vi "poumianS.vi"(0 "object in":refnum<class "212format_work.lvclass">, 1 "in":T2, 5 "error in (no error)":errorcluster) -> (14 "object out":refnum<class "212format_work.lvclass">, 15 "out":T1, 19 "error out":errorcluster)   [LabVIEW 2016, in "212format_work.lvclass"]
uses:
  212format_work.lvclass
  212format_work.lvclass/212format_work.ctl
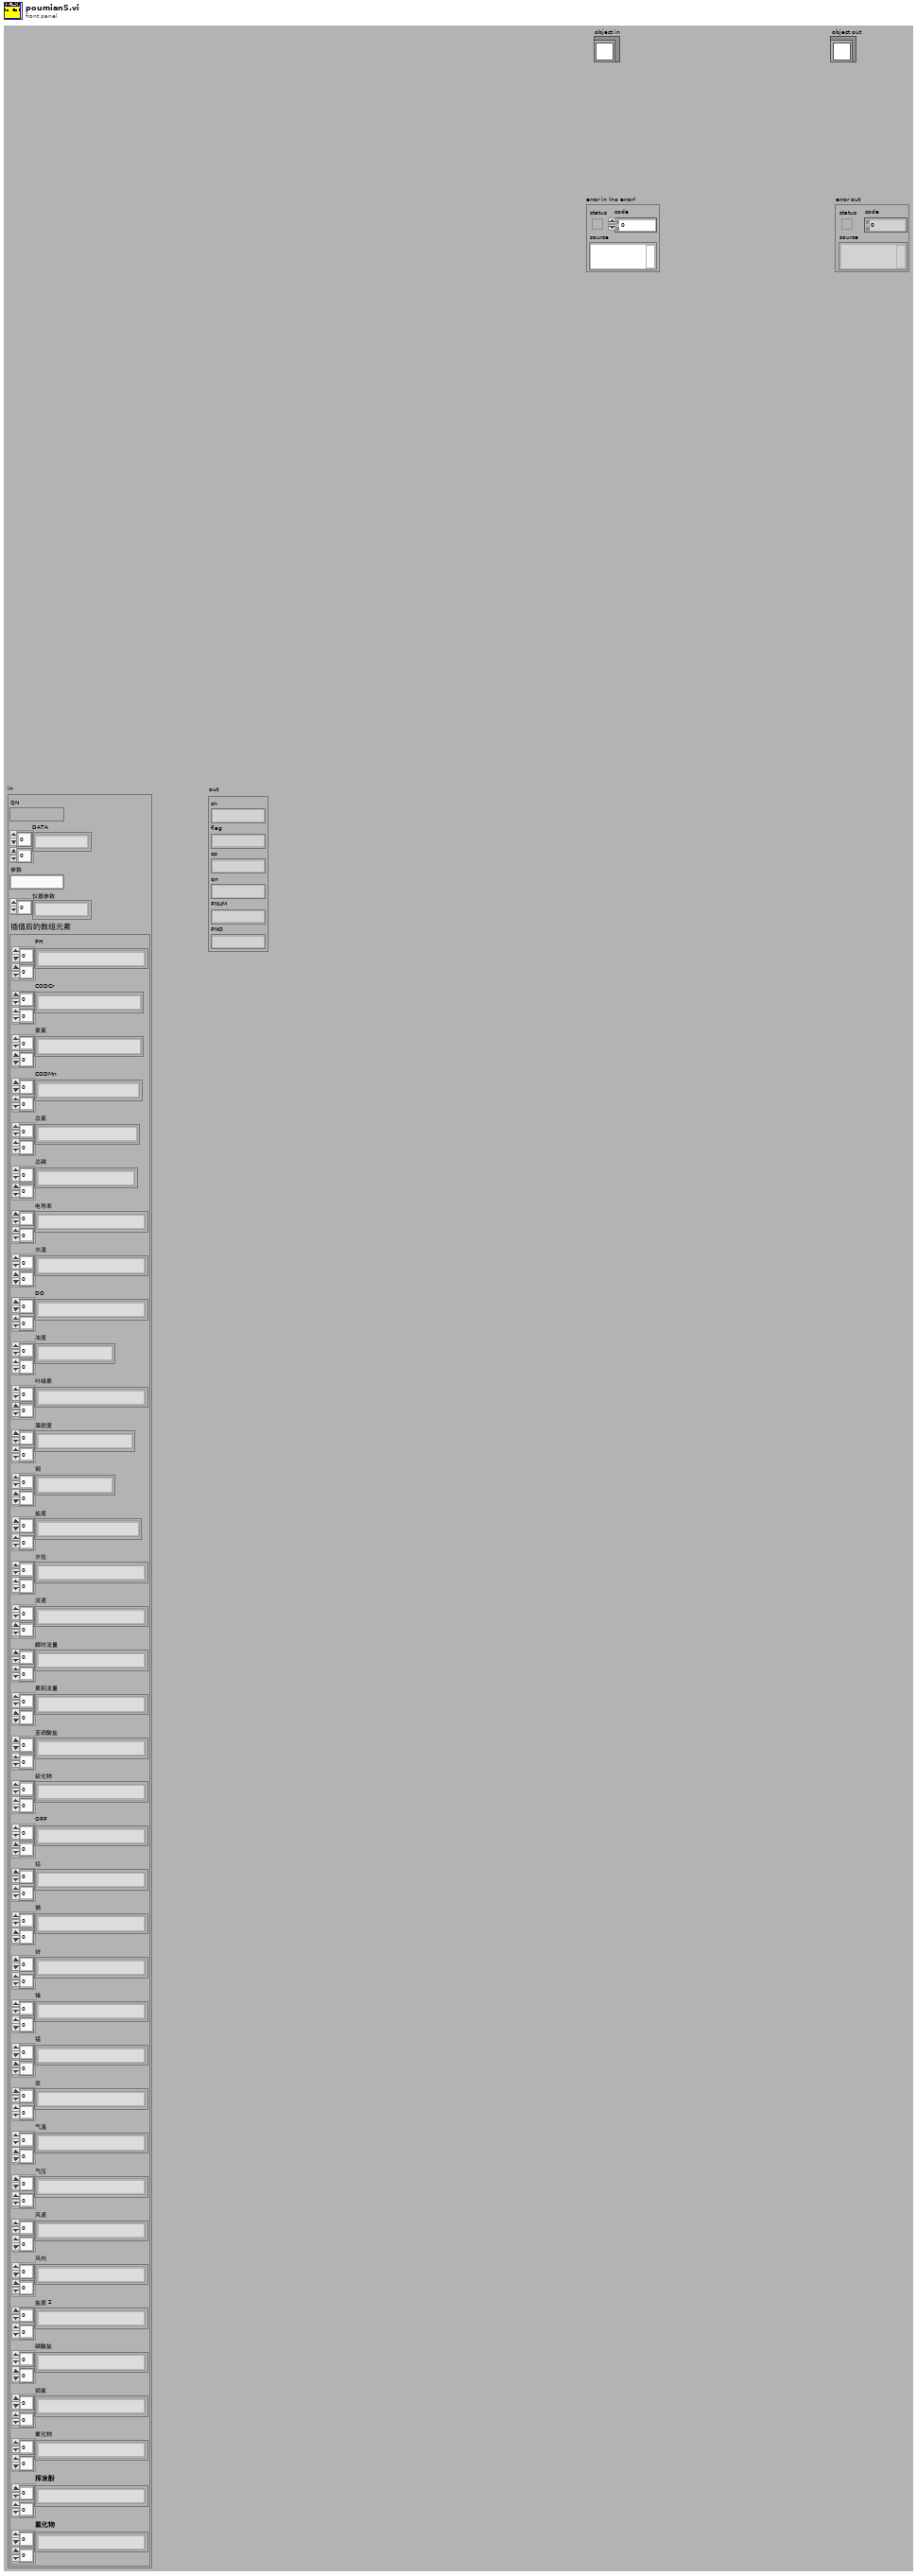
[diagram p1: front panel]
types:
  T1 = cluster{"cn":string, "flag":string, "cp":string, "qn":string, "PNUM":string, "PNO":string}
  T2 = cluster{"QN":string, "DATA":string[][], "参数":string, "仪器参数":string[], "插值后的数组元素":cluster{"PH":string[][], "CODCr":string[][], "氨氮":string[][], "CODMn":string[][], "总氮":string[][], "总磷":string[][], "电导率":string[][], "水温":string[][], "DO":string[][], "浊度":string[][], "叶绿素":string[][], "藻密度":string[][], "铜":string[][], "盐度":string[][], "水位":string[][], "流速":string[][], "瞬时流量":string[][], "累积流量":string[][], "亚硝酸盐":string[][], "硫化物":string[][], "ORP":string[][], "铅":string[][], "镉":string[][], "锌":string[][], "镍":string[][], "锰":string[][], "汞":string[][], "气温":string[][], "气压":string[][], "风速":string[][], "风向":string[][], "盐度 2":string[][], "磷酸盐":string[][], "硝氮":string[][], "氟化物":string[][], "挥发酚":string[][], "氯化物":string[][]}}
  T3 = enum16{"formattime", "formatminute", "formathour"}
  T4 = typedef "212format_work.lvclass/interdata控件.ctl" = cluster{"数据发送协议":enum16{"2005-212协议", "2017-212协议"}, "枚举":enum16{"返回请求应答", "上传数据", "返回执行结果"}, "系统编码ST":string, "主动上报数据中":bool, "数据组合发送":bool, "地表水/污染源":bool, "应用环境":enum16{"STD", "GB212"}}
  T5 = typedef "212format_work.lvclass/data控件.ctl" = cluster{"选择发送的参数":string, "插值后的数组元素":cluster{"PH":string[][], "CODCr":string[][], "氨氮":string[][], "CODMn":string[][], "总氮":string[][], "总磷":string[][], "电导率":string[][], "水温":string[][], "DO":string[][], "浊度":string[][], "叶绿素":string[][], "藻密度":string[][], "铜":string[][], "盐度":string[][], "水位":string[][], "流速":string[][], "瞬时流量":string[][], "累积流量":string[][], "亚硝酸盐":string[][], "硫化物":string[][], "ORP":string[][], "铅":string[][], "镉":string[][], "锌":string[][], "镍":string[][], "锰":string[][], "汞":string[][], "气温":string[][], "气压":string[][], "风速":string[][], "风向":string[][], "盐度 2":string[][], "磷酸盐":string[][], "硝氮":string[][], "氟化物":string[][], "挥发酚":string[][], "氯化物":string[][]}, "register values":u16[], "columns输出":string[], "环境参数":string[][], "仪器编码":string, "实时数据发送间隔":u32, "实时数据参数":string, "参数系数簇":cluster{"CODMn":dbl, "CODCr":dbl, "DO":dbl, "铜":dbl, "PH":dbl, "氨氮":dbl, "比电导率":dbl, "水温":dbl, "COD":dbl, "浊度":dbl, "总氮":dbl, "总磷":dbl, "叶绿素a":dbl, "藻密度":dbl, "水位":dbl, "流速":dbl, "瞬时流量":dbl, "累积流量":dbl, "亚硝酸盐":dbl, "硫化物":dbl, "ORP":dbl, "铅":dbl, "镉":dbl, "锌":dbl, "镍":dbl, "锰":dbl, "汞":dbl, "气温":dbl, "气压":dbl, "风速":dbl, "风向":dbl, "盐度":dbl, "磷酸盐":dbl, "硝氮":dbl, "氟化物":dbl, "挥发酚":dbl, "氯化物":dbl}, "因子编码簇":cluster{"CODMn":string, "CODCr":string, "DO":string, "铜":string, "PH":string, "氨氮":string, "比电导率":string, "水温":string, "COD":string, "浊度":string, "总氮":string, "总磷":string, "叶绿素a":string, "藻密度":string, "水位":string, "流速":string, "瞬时流量":string, "累积流量":string, "亚硝酸盐":string, "硫化物":string, "ORP":string, "铅":string, "镉":string, "锌":string, "镍":string, "锰":string, "汞":string, "气温":string, "气压":string, "风速":string, "风向":string, "盐度":string, "磷酸盐":string, "硝氮":string, "氟化物":string, "挥发酚":string, "氯化物":string}, "小时数据发送次数":i32, "读取试剂余量的值":u16[], "参数编码":string, "数据数组大小":i32, "总包数":i32, "当前包号":i32, "columns":string[], "剖面多参数":string[][], "分包标准":i32}
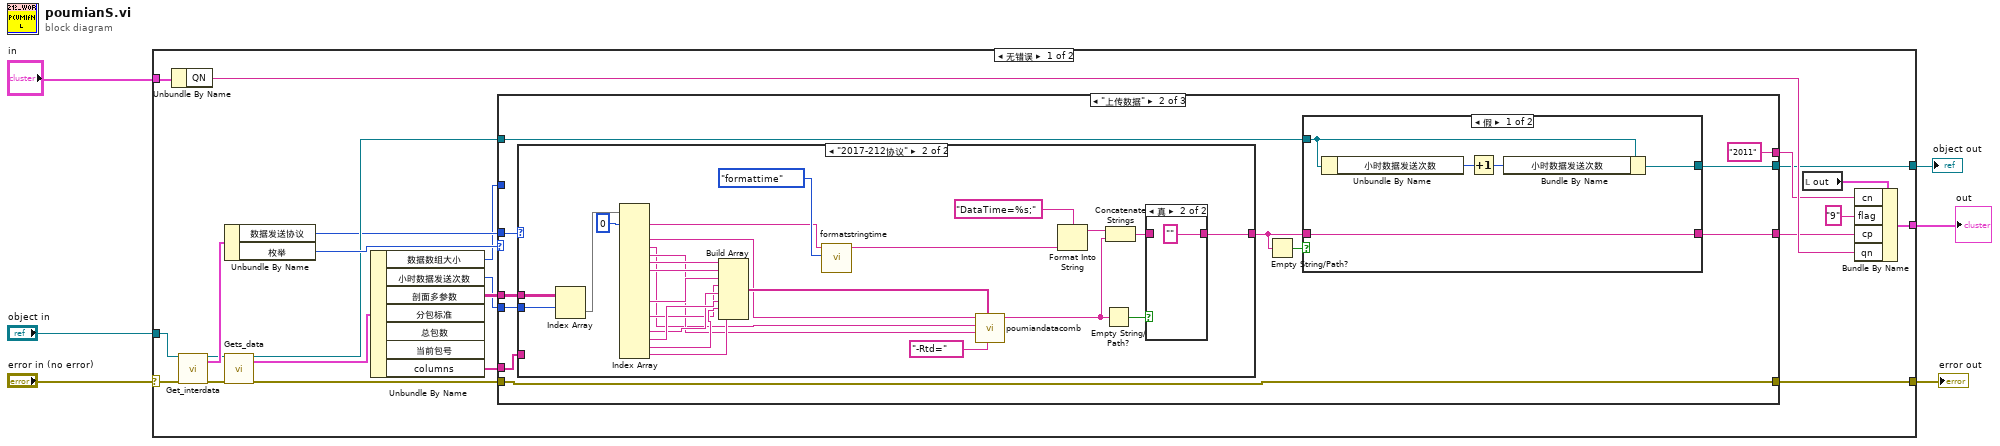
[diagram p0: block diagram]
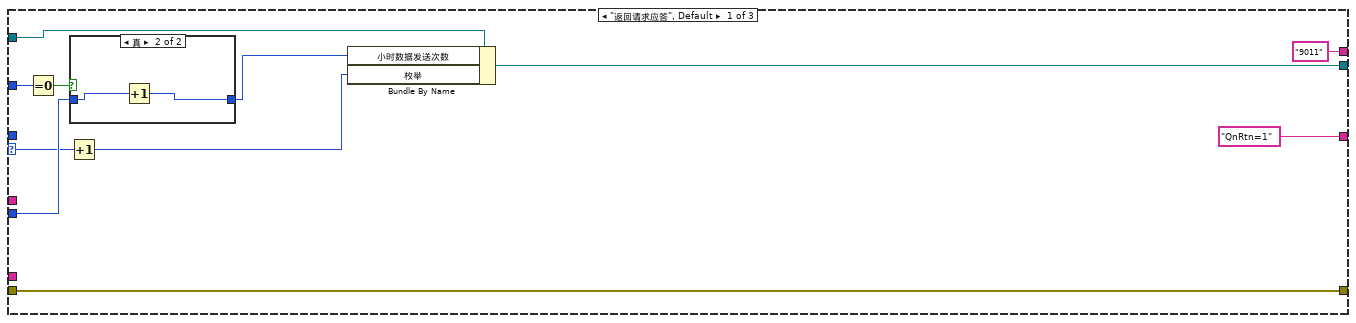
[diagram p2: hidden frame]
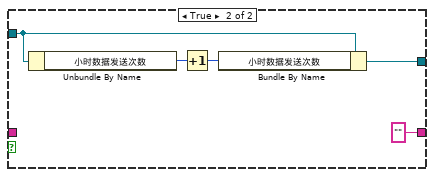
[diagram p4: hidden frame]
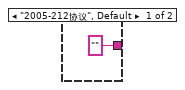
[diagram p5: hidden frame]
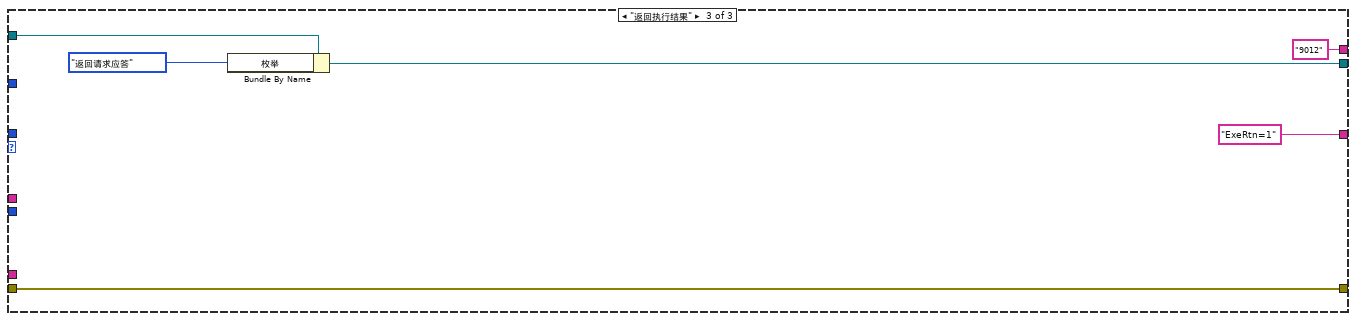
[diagram p7: hidden frame]
diagram:
  n1 = case shown="无错误" "error in (no error)" {
    selector: "error in (no error)" -> [w11 w101]
    tunnel: [w9 w101] -> w5
    tunnel: [w10 w100] -> w3
    tunnel: "object in" -> [w12 w100]
    tunnel: [w8 _] -> w2
    tunnel: "in" -> [w7 _]
    frame No Error {
      n2 = Unbundle By Name(w7) -> ("QN"=w28:string)
      n3 = call-dynamic "Get_interdata.vi"("object in"=w12, "error in (no error)"=w11) -> ("object out"=w22:refnum<class "212format_work.lvclass">, "interdata"=w24:T4, "error out"=w21:errorcluster)  [unwired: 15 in]
      n4 = Unbundle By Name(w24) -> ("数据发送协议"=w15:enum16{"2005-212协议", "2017-212协议"}, "枚举"=w23:enum16{"返回请求应答", "上传数据", "返回执行结果"})
      n5 = call-dynamic "Gets_data.vi"("object in"=w22, "error in (no error)"=w21) -> ("object out"=w17:refnum<class "212format_work.lvclass">, "data"=w20:T5, "error out"=w16:errorcluster)  [unwired: 15 in]
      n6 = Unbundle By Name(w20) -> ("数据数组大小"=w13:i32, "小时数据发送次数"=w18:i32, "剖面多参数"=w19:string[][], "columns"=w14:string[])  [unwired: 3 out]
      n7 = case shown="\"上传数据\"" w23 {
        selector: w23 -> [w34 _ _]
        tunnel: ["9011" ("CN") "2011" ("CN") "9012" ("CN")] -> w27
        tunnel: ["QnRtn=1" w44 "ExeRtn=1"] -> w25
        tunnel: w17 -> [w38 w46 w97]
        tunnel: w19 -> [_ w51 _]
        tunnel: w18 -> [w36 w53 _]
        tunnel: [w32 w45 w95] -> w10
        tunnel: w16 -> [w31 w49 w94]
        tunnel: [w31 w49 w94] -> w9
        tunnel: w15 -> [_ w52 _]
        tunnel: w14 -> [_ w50 _]
        tunnel: w13 -> [w30 _ _]
        frame "返回请求应答", Default {
          n8 = Equal To 0?(x=w30) -> (x = 0?=w37:bool)
          n9 = Increment(x=w34) -> (x+1=w33:enum16{"返回请求应答", "上传数据", "返回执行结果"})
          n10 = case shown="真" w37 {
            tunnel: w36 -> [w41 w43]
            tunnel: [w41 w42] -> w35
            frame False {
            }
            frame True {
              n11 = Increment(x=w43) -> (x+1=w42:i32)
            }
          }
          n12 = Bundle By Name(cluster=w38, "小时数据发送次数"=w35, "枚举"=w33) -> (w32:refnum<class "212format_work.lvclass">)
        }
        frame "上传数据" {
          n13 = case shown="\"2017-212协议\"" w52 {
            tunnel: w53 -> [_ w67]
            tunnel: ["" ("编码输出") w66] -> w47
            tunnel: w51 -> [_ w68]
            tunnel: w50 -> [_ _]
            frame "2005-212协议", Default {
            }
            frame "2017-212协议" {
              n14 = Index Array(array=w68, index (row)=w67) -> (element=w70:string[])  [unwired: 1 in]
              n15 = Index Array(array=w70, index #1=0 ("索引")) -> (element #1=w85:string, element #3=w71:string, element #4=w72:string, element #5=w73:string, element #6=w74:string, element #7=w75:string, element #11=w77:string, element #13=w78:string, element #15=w79:string, element #16=w80:string, element #17=w81:string, element #18=w90:string)  [unwired: 17 in, 6 out]
              n16 = Build Array(w74, w75, w77, w78, w79, w80, w81, w90) -> (w76:string[])
              n17 = call "formatstringtime.vi"("枚举"=T3."formattime", "字符串"=w85) -> ("result string"=w84:string)  [unwired: 9 in]
              n18 = call "poumiandatacomb.vi"("数据类型实时小时"="-Rtd=", "数据值"=w76, "层数"=w73, "数据标识"=w72, "数据类型"=w71) -> ("编码输出"=w88:string)  [unwired: 6 in]
              n19 = Format Into String(format string="DataTime=%s;", w84) -> (resulting string=w83:string)  [unwired: 2 in, 1 out]
              n20 = Empty String/Path?(string/path=w88) -> (empty?=w86:bool)
              n21 = Concatenate Strings(w83, w88) -> (w87:string)
              n22 = case shown="真" w86 {
                tunnel: [w92 ""] -> w66
                tunnel: w87 -> [w92 _]
                frame False {
                }
                frame True {
                }
              }
            }
          }
          n23 = Empty String/Path?(string/path=w47) -> (empty?=w48:bool)
          n24 = case shown="假" w48 {
            tunnel: [w59 ""] -> w44
            tunnel: w47 -> [w59 _]
            tunnel: w46 -> [w58 w61]
            tunnel: [w55 w62] -> w45
            frame False {
              n25 = Unbundle By Name(w58) -> ("小时数据发送次数"=w57:i32)
              n26 = Increment(x=w57) -> (x+1=w56:i32)
              n27 = Bundle By Name(cluster=w58, "小时数据发送次数"=w56) -> (w55:refnum<class "212format_work.lvclass">)
            }
            frame True {
              n28 = Unbundle By Name(w61) -> ("小时数据发送次数"=w60:i32)
              n29 = Increment(x=w60) -> (x+1=w63:i32)
              n30 = Bundle By Name(cluster=w61, "小时数据发送次数"=w63) -> (w62:refnum<class "212format_work.lvclass">)
            }
          }
        }
        frame "返回执行结果" {
          n31 = Bundle By Name(cluster=w97, "枚举"=enum16{"返回请求应答", "上传数据", "返回执行结果"}."返回请求应答" ("interdata.枚举")) -> (w95:refnum<class "212format_work.lvclass">)
        }
      }
      n32 = local read "out"() -> (w29:T1)
      n33 = Bundle By Name(cluster=w29, "cn"=w27, "flag"="9" ("ST"), "cp"=w25, "qn"=w28) -> (w8:T1)
    }
    frame Error {
    }
  }
  "error out" <- w5
  "object out" <- w3
  "out" <- w2
